vi "Init_Images.vi"(8 "error in (no error)":errorcluster, 11 "input cluster in":T1={"Mode"=enum."ROI", "Manual LUT"={"Minimum"=0.0, "Maximum"=0.0}, "ImageProcessed"=refnum, "Image "=refnum, "Log?"=FALSE, "Auto?"=FALSE, "ROI"={"Global Rectangle"=[], "Contours"=[]}, "ROI Parameters"={"Count"=0.0, "Size(um)"=0.0}, "Image X"=0, "Image Y"=0, "Horizontal ROI"={"Global Rectangle"=[], "Contours"=[]}, "HROI Pos"=0, "Custom ROI"={"Global Rectangle"=[], "Contours"=[]}, "Intensity Graph"=[], "Image Type"=7, "ImagePreview"=refnum} {"Image Type" items=["Grayscale (U8)", "Grayscale (U16)"]; "ROI Parameters"."Size(um)" min=0 max=255 step=0.1 format="%.2f"; "ROI Parameters"."Count" min=0 max=255 step=0.1 format="%.2f"}) -> (0 "error out":errorcluster, 1 "input cluster out":T1={"Mode"=enum."ROI", "Manual LUT"={"Minimum"=0.0, "Maximum"=0.0}, "ImageProcessed"=refnum, "Image "=refnum, "Log?"=FALSE, "Auto?"=FALSE, "ROI"={"Global Rectangle"=[], "Contours"=[]}, "ROI Parameters"={"Count"=0.0, "Size(um)"=0.0}, "Image X"=0, "Image Y"=0, "Horizontal ROI"={"Global Rectangle"=[], "Contours"=[]}, "HROI Pos"=0, "Custom ROI"={"Global Rectangle"=[], "Contours"=[]}, "Intensity Graph"=[], "Image Type"=7, "ImagePreview"=refnum} {"Image Type" items=["Grayscale (U8)", "Grayscale (U16)"]; "ROI Parameters"."Size(um)" min=0 max=255 step=0.1 format="%.2f"; "ROI Parameters"."Count" min=0 max=255 step=0.1 format="%.2f"}, 5 "Image Pixels (U8)":u8[][](array[numeric]))   [LabVIEW 2023, in "Camera_Controller.lvlib" / "Camera_Controller.lvclass"]
uses:
  Camera_Controller.lvclass
  typedefs/ImageProcessingParameters.ctl
  <vilib>/vision/Image Controls.llb/IMAQ Image.ctl
  typedefs/Image Type.ctl
  Camera_Controller.lvclass/Camera_Controller.ctl
  typedefs/typedefs.lvlib
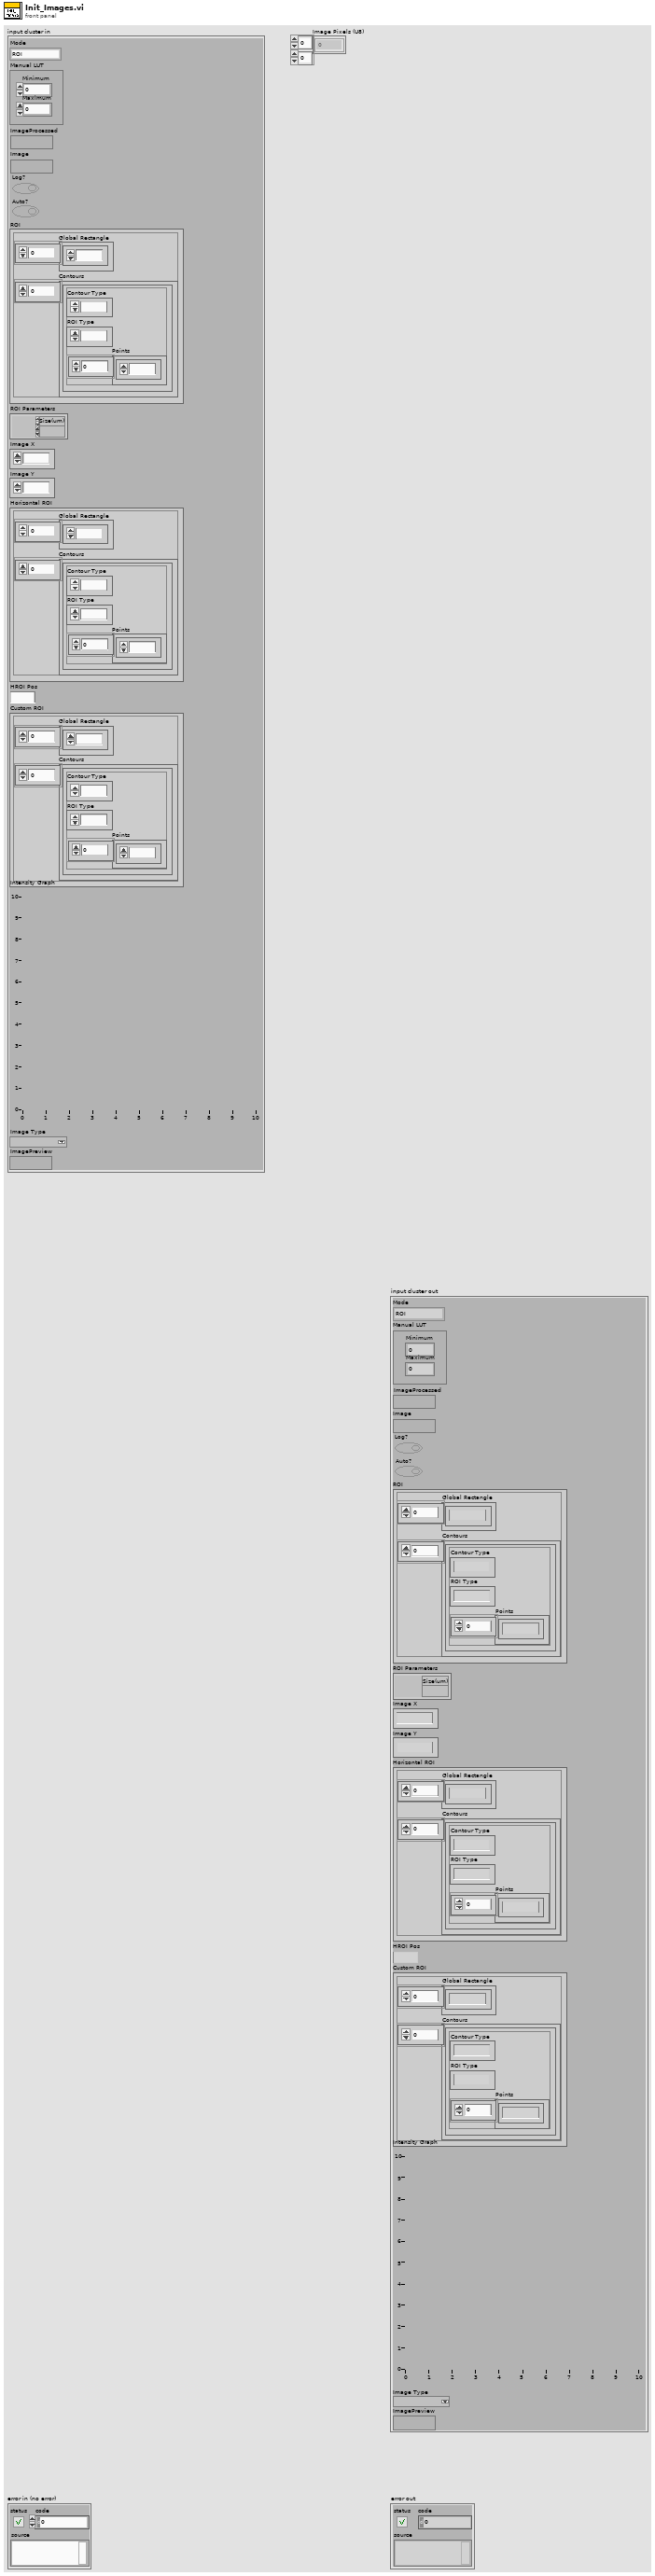
[diagram p1: front panel]
types:
  T1 = typedef "typedefs.lvlib/ImageProcessingParameters.ctl" = cluster{"Mode":enum16{"ROI", "Image"}, "Manual LUT":cluster{"Minimum":dbl, "Maximum":dbl}, "ImageProcessed":T2, "Image ":T2, "Log?":bool, "Auto?":bool, "ROI":cluster{"Global Rectangle":i32[], "Contours":cluster{"Contour Type":u32, "ROI Type":u32, "Points":i32[]}[]}, "ROI Parameters":cluster{"Count":sgl, "Size(um)":sgl}, "Image X":i32, "Image Y":i32, "Horizontal ROI":cluster{"Global Rectangle":i32[], "Contours":cluster{"Contour Type":u32, "ROI Type":u32, "Points":i32[]}[]}, "HROI Pos":u16, "Custom ROI":cluster{"Global Rectangle":i32[], "Contours":cluster{"Contour Type":u32, "ROI Type":u32, "Points":i32[]}[]}, "Intensity Graph":u8[][], "Image Type":T3, "ImagePreview":T2}
  T2 = typedef "IMAQ Image.ctl" = refnum<image>
  T3 = typedef "typedefs.lvlib/Image Type.ctl" = u32
  T4 = typedef "Image Type" = u32
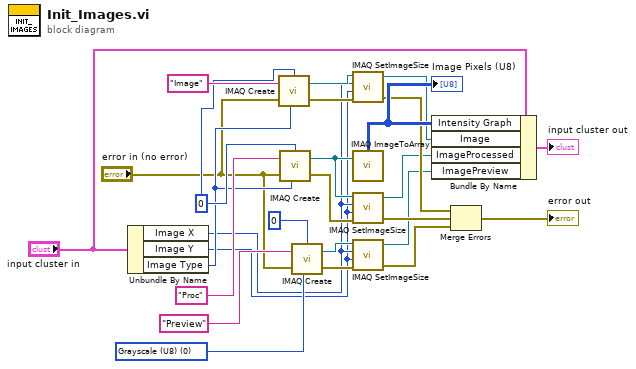
[diagram p0: block diagram]
diagram:
  w10 = T4 0 items=["Grayscale (U8)", "Grayscale (I16)", "Grayscale (SGL)", "Complex (CSG)", "RGB (U32)", "HSL (U32)", "RGB (U64)", "Grayscale (U16)"] ("Image Type")
  w12 = 0 ("Border Size")
  n1 = Unbundle By Name("input cluster in") -> ("Image X"=w3:i32, "Image Y"=w2:i32, "Image Type"=w11:T3)
  n2 = call "IMAQ Create"("Border Size"=w12, "Image Name"="Image", "Image Type"=w11, "error in (no error)"="error in (no error)") -> ("New Image"=w18:T2, "error out"=w22:errorcluster)  [unwired: 1 in]
  n3 = call "IMAQ Create"("Border Size"=w12, "Image Name"="Proc", "Image Type"=w11, "error in (no error)"="error in (no error)") -> ("New Image"=w25:T2, "error out"=w20:errorcluster)  [unwired: 1 in]
  n4 = call "IMAQ Create"("Border Size"=0, "Image Name"="Preview", "Image Type"=w10, "error in (no error)"="error in (no error)") -> ("New Image"=w8:T2, "error out"=w6:errorcluster)  [unwired: 1 in]
  n5 = call "IMAQ SetImageSize"("error in (no error)"=w22, "Y Resolution"=w2, "X Resolution"=w3, "Image"=w18) -> ("error out"=w23:errorcluster, "Image Out"=w24:T2)  [unwired: 1 in]
  n6 = call "IMAQ ImageToArray"("Image"=w25) -> ("Image Pixels (U8)"=w26:u8[][])  [unwired: 3 in, 4 out]
  "Image Pixels (U8)" <- w26
  n7 = call "IMAQ SetImageSize"("error in (no error)"=w20, "Y Resolution"=w2, "X Resolution"=w3, "Image"=w25) -> ("error out"=w21:errorcluster, "Image Out"=w19:T2)  [unwired: 1 in]
  n8 = call "IMAQ SetImageSize"("error in (no error)"=w6, "Y Resolution"=w2, "X Resolution"=w3, "Image"=w8) -> ("error out"=w4:errorcluster, "Image Out"=w1:T2)  [unwired: 1 in]
  n9 = Bundle By Name(cluster="input cluster in", "Intensity Graph"=w26, "Image"=w24, "ImageProcessed"=w19, "ImagePreview"=w1) -> (→"input cluster out":T1)
  n10 = Merge Errors(w23, w21, w4) -> (→"error out":errorcluster)
